vi "Camera Process.vi"(0 "error in":errorcluster) -> ()   [LabVIEW 2012]
uses:
  Camera Global Data.vi
  BotStatus.vi
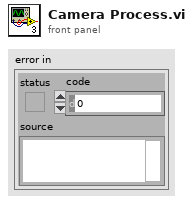
[diagram p1: front panel]
types:
  T1 = cluster{"Y Axis":dbl, "X Axis":dbl, "View Ground":bool, "Center On Target":bool, "Stop Auto move?":bool, "Servo X Current":dbl, "Servo Y Current":dbl, "Target Info":cluster{"Target Found?":bool, "Target X Position":dbl, "Target Y Position":dbl}, "Seen Floor X Angle":dbl, "Seen Floor Y Angle":dbl, "Centerd?":bool, "Servo X Set":dbl, "Servo Y Set":dbl}
  T2 = cluster{"Target Position X":dbl, "Target Position Y":dbl, "Target Found":bool}
  T3 = cluster{"Target Found?":bool, "Target X Position":dbl, "Target Y Position":dbl}
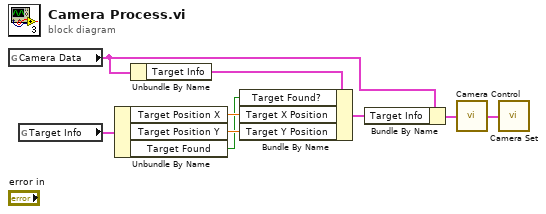
[diagram p0: block diagram]
diagram:
  n1 = global read "Camera Global Data.vi" "Camera Data"() -> (w7:T1)
  n2 = global read "BotStatus.vi" "Target Info"() -> (w4:T2)
  n3 = Unbundle By Name(w4) -> ("Target Position X"=w3:dbl, "Target Position Y"=w2:dbl, "Target Found"=w1:bool)
  n4 = Unbundle By Name(w7) -> ("Target Info"=w6:T3)
  n5 = Bundle By Name(cluster=w6, "Target Found?"=w1, "Target X Position"=w3, "Target Y Position"=w2) -> (w5:T3)
  n6 = Bundle By Name(cluster=w7, "Target Info"=w5) -> (w8:T1)
  n7 = call "Camera Control.vi"("Camera Data"=w8) -> ("Camera Data out"=w9:T1)
  n8 = call "Camera Set.vi"("Camera Data"=w9) -> ()
